vi "Time Since Called.vi"(1 "Reset":bool) -> (0 "Numeric":dbl)   [LabVIEW 2019]
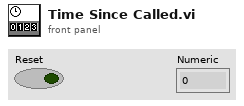
[diagram p1: front panel]
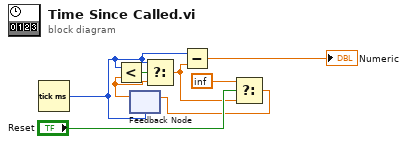
[diagram p0: block diagram]
diagram:
  n1 = Tick Count (ms)() -> (millisecond timer value=w1:u32)
  n2 = feedback #1(w1) -> (w3:dbl)
  n3 = Less?(x=w1, y=w3) -> (x < y?=w2:bool)
  n4 = Select(t=w1, s=w2, f=w3) -> (s? t:f=w5:dbl)
  n5 = Subtract(x=w1, y=w5) -> (x-y=→"Numeric":dbl)
  n6 = Select(t=inf, s="Reset", f=w5) -> (s? t:f=w6:dbl)
  n7 = feedback-in #1(w6) -> ()
